vi "wait on clock.vi"(8 "error in":errorcluster, 10 "dt":u32=1, 11 "timing source in":refnum<class "TBM timing source.lvclass">) -> (0 "error out":errorcluster, 2 "ticks since last call":u32, 3 "timing source out":refnum<class "TBM timing source.lvclass">)   [LabVIEW 2013, in "TBM timing source.lvclass"]
doc: "This core timing function is used inside of a loop to wait for a clock signal, or dt ticks of a clock signal."
uses:
  TBM timing source.lvclass
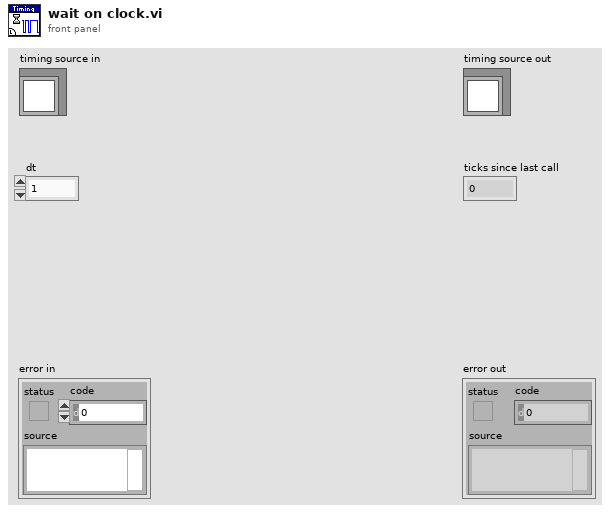
[diagram p1: front panel]
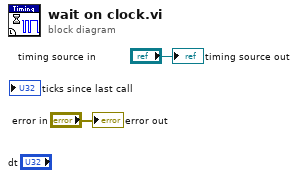
[diagram p0: block diagram]
diagram:
  "error out" <- "error in"
  "timing source out" <- "timing source in"
